vi "getActorName.vi"(8 "error in":errorcluster, 9 "Actor Names":string[](array[string]), 10 "axis in":u8, 11 "connection ID":refnum<k5>) -> (0 "error out":errorcluster, 1 "ActorName out":string, 2 "axis out":u8, 3 "connection ID":refnum<k5>)   [LabVIEW 2016]
panel:
  in  "Get Command":string="com.attocube.amc.control.getActorName"
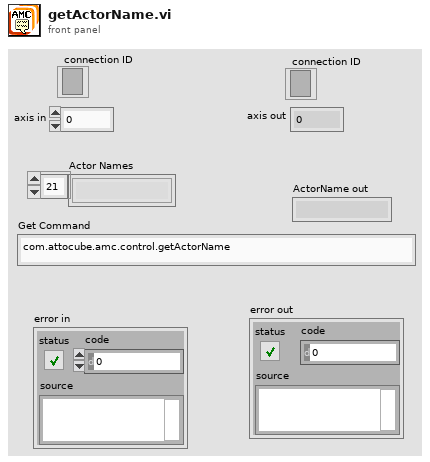
[diagram p1: front panel]
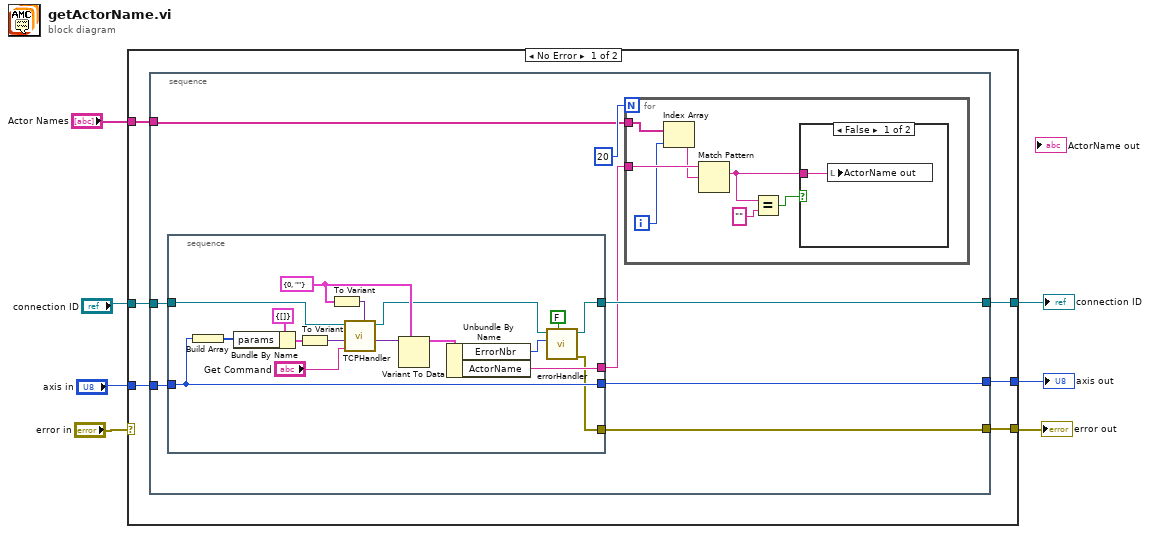
[diagram p0: block diagram]
diagram:
  n1 = case shown="No Error" "error in" {
    selector: "error in" -> [_ w49]
    tunnel: "axis in" -> [w13 w48]
    tunnel: [w12 w49] -> w6
    tunnel: [w11 w48] -> w5
    tunnel: "connection ID" -> [w10 w47]
    tunnel: "Actor Names" -> [w9 _]
    tunnel: [w8 w47] -> w1
    frame No Error {
      n2 = stacked-sequence {
        tunnel: w13 -> [w18]
        tunnel: [w17] -> w11
        tunnel: [w15] -> w12
        tunnel: w10 -> [w14]
        tunnel: w9 -> [w20]
        tunnel: [w19] -> w8
        frame #0 {
          n3 = stacked-sequence {
            tunnel: [w26] -> w19
            tunnel: w14 -> [w31]
            tunnel: [w28] -> w16
            tunnel: w18 -> [w25]
            tunnel: [w25] -> w17
            tunnel: [w23] -> w15
            frame #0 {
              w29 = cluster{"ErrorNbr":i32, "ActorName":string} {"ErrorNbr"=0, "ActorName"=""} ("input cluster")
              n4 = Build Array(w25) -> (w35:u8[])
              n5 = Bundle By Name(cluster=cluster{"params":i16[]} {"params"=[]} ("input cluster"), "params"=w35) -> (w36:cluster{"params":i16[]})
              n6 = To Variant(anything=w36) -> (Variant=w37:variant)
              n7 = To Variant(anything=w29) -> (Variant=w30:variant)
              n8 = call "TCPHandler.vi"("result Types"=w30, "method"="Get Command", "params"=w37, "connection ID"=w31) -> ("result"=w33:variant, "connection ID"=w27:refnum<k5>)  [unwired: 5 in, 1 out]
              n9 = Variant To Data(type=w29, Variant=w33) -> (data=w38:cluster{"ErrorNbr":i32, "ActorName":string})  [unwired: 1 in, 1 out]
              n10 = Unbundle By Name(w38) -> ("ErrorNbr"=w22:i32, "ActorName"=w28:string)
              n11 = call "errorHandler.vi"("show popup"=FALSE, "error number"=w22, "connection ID"=w27) -> ("error out"=w23:errorcluster, "connection ID"=w26:refnum<k5>)  [unwired: 7 in]
            }
          }
          n12 = for {
            N: 20 -> [_]
            tunnel: w16 -> [w45]
            tunnel: w20 -> [w42]
            i -> [w44]
            n13 = Index Array(array=w42, index=w44) -> (element=w43:string)
            n14 = Match Pattern(string=w45, regular expression=w43) -> (match substring=w39:string)  [unwired: 1 in, 3 out]
            n15 = Equal?(x=w39, y="") -> (x = y?=w40:bool)
            n16 = case shown="False" w40 {
              tunnel: w39 -> [w46 _]
              frame False {
                n17 = local write "ActorName out"(w46) -> ()
              }
              frame True {
              }
            }
          }
        }
      }
    }
    frame Error {
    }
  }
  "error out" <- w6
  "axis out" <- w5
  "connection ID" <- w1
